vi "Add Tree Nodes.vi"(7 "Root path":string, 8 "Event Types":T1[](array[typedef]), 9 "map ref in":map{string, refnum<vi>}(c390), 10 "DQMH Lib In":refnum<vi>, 11 "Tree Map in":T2) -> (1 "map ref out":map{string, refnum<vi>}(c390), 3 "Tree Map out":T2)   [LabVIEW 2020, in "Panter Dashboard.lvlib"]
uses:
  Panter Dashboard.lvlib
  <vilib>/National Instruments/Tree Map/Tree Map Data.ctl
  Event types--enum.ctl
  <vilib>/Delacor/Delacor QMH/Libraries/Scripting API/DQMH_Scripting API.lvlib
  <vilib>/National Instruments/Tree Map/Tree Map.lvlib
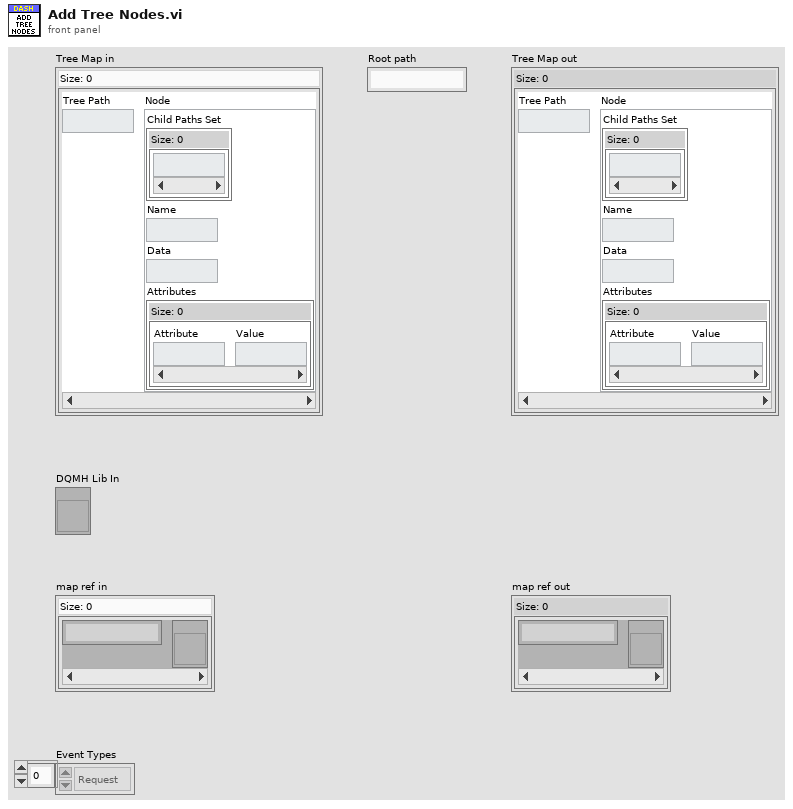
[diagram p1: front panel]
types:
  T1 = typedef "Panter Dashboard.lvlib/Event types--enum.ctl" = enum16{"Request", "Request and Wait for Reply", "Broadcast"}
  T2 = typedef "Tree Map.lvlib/Tree Map Data.ctl" = map{string, cluster{"Child Paths Set":set{string}, "Name":string, "Data":string, "Attributes":map{string, string}}}
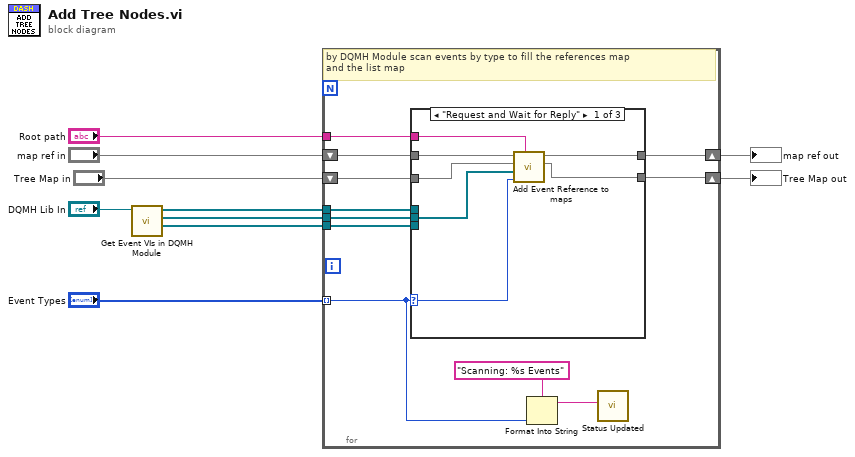
[diagram p0: block diagram]
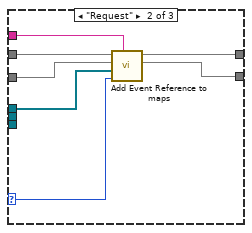
[diagram p2: hidden frame]
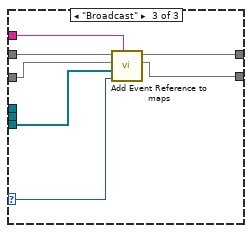
[diagram p3: hidden frame]
diagram:
  n1 = call <vilib>:"Get Event VIs in DQMH Module.vi"("DQMH Module"="DQMH Lib In") -> ("Broadcast Event VIs"=w1:refnum<vi>[], "Request and Wait for Reply Event VIs"=w2:refnum<vi>[], "Request Event VIs"=w3:refnum<vi>[])  [unwired: 7 in, 1 out]
  n2 = for {
    tunnel: "Root path" -> [w15]
    tunnel: "Event Types" -> [w12] mode=indexing
    shift-right: [w21] -> w10
    shift-left: "map ref in" -> [w20]
    shift-right: [w19] -> w7
    shift-left: "Tree Map in" -> [w14]
    tunnel: w3 -> [w18]
    tunnel: w2 -> [w17]
    tunnel: w1 -> [w16]
    # "by DQMH Module scan events by type to fill the references map\nand the list map"
    n3 = case shown="\"Request and Wait for Reply\"" w12 {
      selector: w12 -> [w23 w31 w38]
      tunnel: [w28 w35 w42] -> w21
      tunnel: w20 -> [w27 w34 w41]
      tunnel: [w26 w33 w40] -> w19
      tunnel: w18 -> [_ w29 _]
      tunnel: w17 -> [w24 _ _]
      tunnel: w16 -> [_ _ w37]
      tunnel: w15 -> [w22 w30 w36]
      tunnel: w14 -> [w25 w32 w39]
      frame "Request and Wait for Reply" {
        n4 = call "Add Event Reference to maps.vi"("New Node Path"=w22, "Event type"=w23, "Event VIs"=w24, "Tree Map in"=w25, "map ref in"=w27) -> ("Tree Map out"=w26:T2, "map ref out"=w28:map{string, refnum<vi>})  [unwired: 5 in]
      }
      frame "Request" {
        n5 = call "Add Event Reference to maps.vi"("New Node Path"=w30, "Event type"=w31, "Event VIs"=w29, "Tree Map in"=w32, "map ref in"=w34) -> ("Tree Map out"=w33:T2, "map ref out"=w35:map{string, refnum<vi>})  [unwired: 5 in]
      }
      frame "Broadcast" {
        n6 = call "Add Event Reference to maps.vi"("New Node Path"=w36, "Event type"=w38, "Event VIs"=w37, "Tree Map in"=w39, "map ref in"=w41) -> ("Tree Map out"=w40:T2, "map ref out"=w42:map{string, refnum<vi>})  [unwired: 5 in]
      }
    }
    n7 = Format Into String(format string="Scanning: %s Events", w12) -> (resulting string=w13:string)  [unwired: 2 in, 1 out]
    n8 = call "Status Updated.vi"("Status"=w13) -> ()  [unwired: 10 in, 1 out]
  }
  "map ref out" <- w10
  "Tree Map out" <- w7
